vi "BRig_dataCurrent_T_Cue.vi"() -> (2 "output_T_Cue":i32)   [LabVIEW 2014]
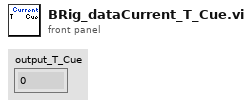
[diagram p1: front panel]
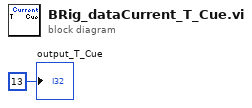
[diagram p0: block diagram]
diagram:
  "output_T_Cue" <- 13 ("output_iBlock")
